vi "get_embed_delta.vi"(8 "error in (no error)":errorcluster, 11 "Canonical IDs":i32[](array[numeric])) -> (0 "error out":errorcluster, 2 "Reference ID":i32, 3 "Embed delta":refnum<queue>)   [LabVIEW 2023]
uses:
  <vilib>/Utility/error.llb/Trim Whitespace One-Sided.vi
  <vilib>/httpClient/LabVIEWHTTPClient.lvlib
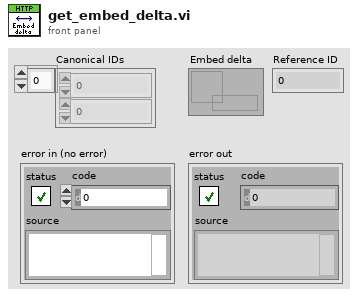
[diagram p1: front panel]
types:
  T1 = typedef "LabVIEWHTTPClient.lvlib/ClientHandle.ctl" = refnum<k1>
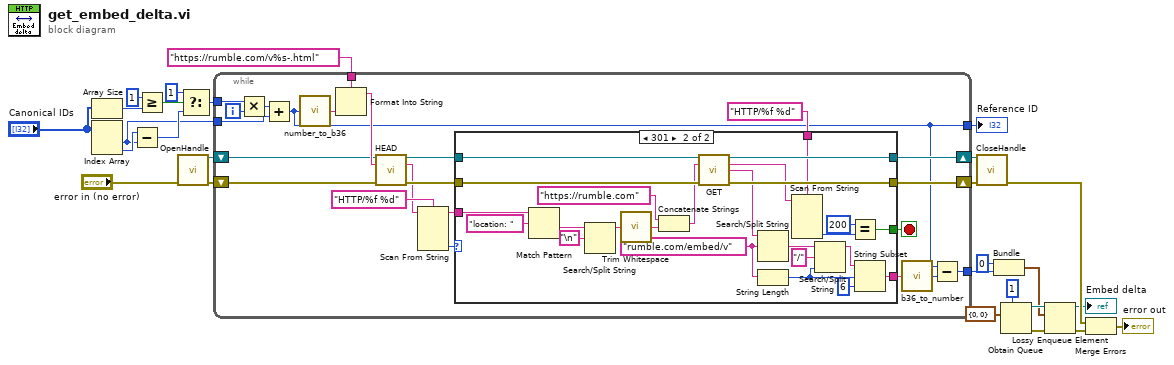
[diagram p0: block diagram]
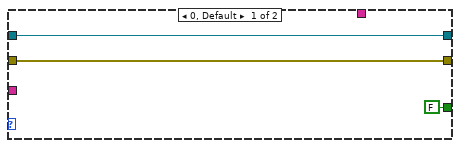
[diagram p2: hidden frame]
diagram:
  n1 = Array Size(array="Canonical IDs") -> (size(s)=w19:i32)
  n2 = Index Array(array="Canonical IDs") -> (element #1=w13:i32, element #2=w21:i32)  [unwired: 2 in]
  n3 = Subtract(x=w21, y=w13) -> (x-y=w15:i32)
  n4 = Greater Or Equal?(x=1, y=w19) -> (x >= y?=w17:bool)
  n5 = call <vilib>:"OpenHandle.vi"("error in (no error)"="error in (no error)") -> ("client handle out"=w26:T1, "error out"=w25:errorcluster)  [unwired: 13 in]
  n6 = Select(t=1 ("x"), s=w17, f=w15) -> (s? t:f=w14:i32)
  n7 = while {
    tunnel: "https://rumble.com/v%s-.html" ("url") -> [w49]
    shift-right: [w40] -> w23
    shift-left: w26 -> [w47]
    shift-right: [w39] -> w22
    shift-left: w25 -> [w46]
    tunnel: w14 -> [w37]
    tunnel: w13 -> [w35]
    tunnel: [w31] -> w10
    tunnel: [w28] -> w12
    i -> [w38]
    stop <- w34 stop-if-true
    n8 = Multiply(x=w37, y=w38) -> (x*y=w36:i32)
    n9 = Add(x=w36, y=w35) -> (x+y=w28:i32)
    n10 = call "number_to_b36.vi"("Number"=w28) -> ("Base36 string"=w48:string)
    n11 = Format Into String(format string=w49, w48) -> (resulting string=w50:string)  [unwired: 2 in, 1 out]
    n12 = call <vilib>:"HEAD.vi"("client handle"=w47, "url"=w50, "error in (no error)"=w46) -> ("client handle out"=w42:T1, "headers"=w30:string, "error out"=w41:errorcluster)  [unwired: 10 in]
    n13 = Scan From String(format string="HTTP/%f %d", input string=w30) -> (remaining string=w43:string, output 2=w44:i32)  [unwired: 5 in, 2 out]
    n14 = case shown="301" w44 {
      tunnel: w43 -> [_ w78]
      tunnel: w42 -> [w53 w73]
      tunnel: w41 -> [w52 w72]
      tunnel: [_ w64] -> w29
      tunnel: [w53 w63] -> w40
      tunnel: [w52 w62] -> w39
      tunnel: [FALSE w57] -> w34
      tunnel: "HTTP/%f %d" ("format string") -> [_ w60]
      frame 0, Default {
      }
      frame 301 {
        w66 = "rumble.com/embed/v" ("search string/char (-)")
        n15 = Match Pattern(string=w78, regular expression="location: ") -> (after substring=w76:string)  [unwired: 1 in, 3 out]
        n16 = Search/Split String(string=w76, search string/char (-)="\n") -> (substring before match=w74:string)  [unwired: 1 in, 2 out]
        n17 = call <vilib>:"Trim Whitespace.vi"("string"=w74) -> ("trimmed string"=w71:string)  [unwired: 1 in]
        n18 = Concatenate Strings("https://rumble.com" ("url"), w71) -> (w55:string)
        n19 = call <vilib>:"GET.vi"("client handle"=w73, "url"=w55, "error in (no error)"=w72) -> ("client handle out"=w63:T1, "headers"=w61:string, "body"=w54:string, "error out"=w62:errorcluster)  [unwired: 9 in]
        n20 = Search/Split String(string=w54, search string/char (-)=w66) -> (match + rest of string=w67:string)  [unwired: 1 in, 2 out]
        n21 = String Length(string=w66) -> (length=w69:i32)
        n22 = Scan From String(format string=w60, input string=w61) -> (output 2=w59:i32)  [unwired: 5 in, 3 out]
        n23 = Search/Split String(string=w67, search string/char (-)="/", offset (0)=w69) -> (substring before match=w68:string)  [unwired: 2 out]
        n24 = Equal?(x=200, y=w59) -> (x = y?=w57:bool)
        n25 = String Subset(string=w68, offset (0)=w69, length (rest)=6 ("length (rest)")) -> (substring=w64:string)
      }
    }
    n26 = call "b36_to_number.vi"("Base36 string"=w29) -> ("Number"=w32:i32)
    n27 = Subtract(x=w28, y=w32) -> (x-y=w31:i32)
  }
  "Reference ID" <- w12
  n28 = call <vilib>:"CloseHandle.vi"("client handle"=w23, "error in (no error)"=w22) -> ("error out"=w2:errorcluster)  [unwired: 13 in]
  n29 = Bundle(0, w10) -> (w6:cluster{i32, i32})  [unwired: 1 in]
  n30 = Obtain Queue(max queue size (-1, unlimited)=1, element data type=cluster{"Index":i32, "Embed delta":i32} {"Index"=0, "Embed delta"=0}) -> (queue out=w7:refnum<queue>, error out=w5:errorcluster)  [unwired: 3 in, 1 out]
  n31 = Lossy Enqueue Element(queue=w7, element=w6, error in (no error)=w5) -> (queue out=→"Embed delta":refnum<queue>, error out=w4:errorcluster)  [unwired: 2 out]
  n32 = Merge Errors(w2, w4) -> (→"error out":errorcluster)
